vi "VI Tree - comparison__ogtk.vi"   [LabVIEW 2011]
uses:
  Variant Changed__ogtk.vi
panel:
  # "[OpenG VI Tags] ***Do Not Remove***"
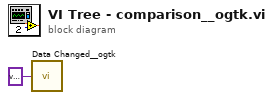
[diagram p0: block diagram]
diagram:
  n1 = call-poly "Data Changed__ogtk.vi"("Variant"=variant) -> ()  [unwired: 1 out]
